vi "Fourier Transform Open VI Final.vi"() -> ()   [LabVIEW 2021]
uses:
  <vilib>/Analysis/4window.llb/windowTd.ctl
  <vilib>/Analysis/4window.llb/Hanning Window (DBL).vi
  <vilib>/Analysis/4window.llb/AllCosWindow (DBL).vi
  <vilib>/Utility/file.llb/Read Delimited Spreadsheet (DBL).vi
  <vilib>/Analysis/2dsp.llb/Zero Padder (DBL).vi
  <vilib>/measure/maspectr.llb/FFT Spectrum (Mag-Phase) for 1 Chan.vi
  <vilib>/measure/NI_MAPro.lvlib
  <vilib>/Analysis/NI_AALPro.lvlib
panel:
  out "Transient":cluster{dbl[], "magnitude":dbl[]}(graph)
  in  "Max m/z Value":dbl=5000.0
  in  "Zero Paddings":i32
  out "Mass Spectrum":cluster{dbl[], "magnitude":dbl[]}(graph)
  out "Mass Calibration Factor":dbl
  out "Frequency (Hz)":dbl
  in  "File Path":path
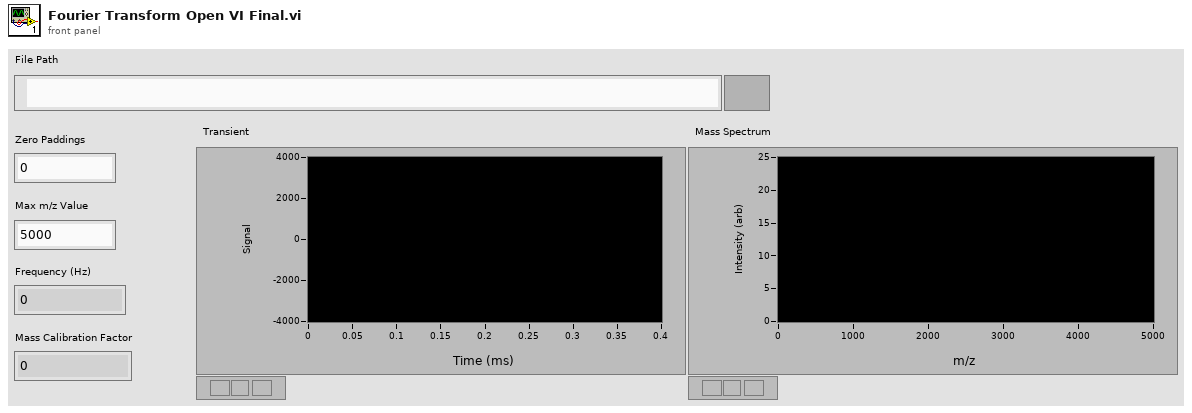
[diagram p1: front panel]
types:
  T1 = typedef "NI_AALPro.lvlib/windowTd.ctl" = u32
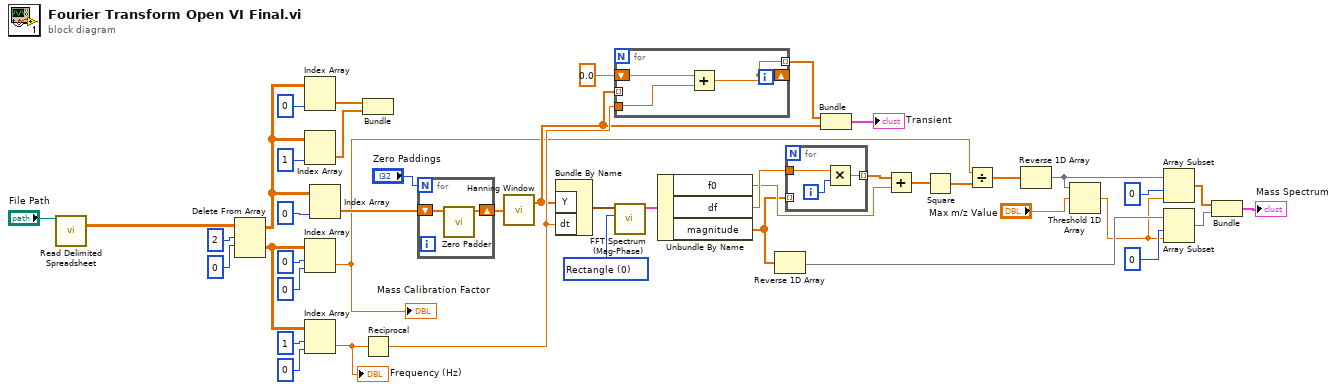
[diagram p0: block diagram]
diagram:
  w26 = T1 0 items=["Rectangle"=0, "Hanning"=1, "Hamming"=2, "Blackman-Harris"=3, "Exact Blackman"=4, "Blackman"=5, "Flat Top"=6, "4 Term B-Harris "=7, "7 Term B-Harris"=8, "Low Sidelobe"=9, "Blackman Nuttall"=11, "Triangle"=30, "Bartlett-Hanning"=31, "Bohman"=32, "Parzen"=33, "Welch"=34, "Kaiser"=60, "Dolph-Chebyshev"=61, "Gaussian"=62] ("window")
  n1 = call-poly <vilib>:"Read Delimited Spreadsheet.vi"("file path (dialog if empty)"="File Path") -> ("all rows"=w43:dbl[][])  [unwired: 9 in, 5 out]
  n2 = Delete From Array(array=w43, length=2, index (row)=0) -> (deleted portion=w39:dbl[][], array with subset deleted=w13:dbl[][])  [unwired: 1 in]
  n3 = Index Array(array=w13, index (col)=0 ("disabled index (col)")) -> (element=w10:dbl[])  [unwired: 1 in]
  n4 = Index Array(array=w13, index (col)=1 ("disabled index (col)")) -> (element=w11:dbl[])  [unwired: 1 in]
  n5 = Index Array(array=w39, index (row)=0, index (col)=0 ("disabled index (col)")) -> (element=w1:dbl)
  "Mass Calibration Factor" <- w1
  n6 = Index Array(array=w39, index (row)=1, index (col)=0 ("disabled index (col)")) -> (element=w29:dbl)
  "Frequency (Hz)" <- w29
  n7 = Index Array(array=w13, index (col)=0 ("disabled index (col)")) -> (element=w32:dbl[])  [unwired: 1 in]
  n8 = Bundle("all rows"=w10, "all rows"=w11) -> ()  [unwired: 1 in, 1 out]
  n9 = Reciprocal(x=w29) -> (1/x=w8:dbl)
  n10 = for {
    N: "Zero Paddings" -> [_]
    shift-right: [w45] -> w31
    shift-left: w32 -> [w46]
    n11 = call-poly <vilib>:"Zero Padder.vi"("Input Array"=w46) -> ("Zero Padded Array"=w45:dbl[])  [unwired: 10 in]
  }
  n12 = call-poly <vilib>:"Hanning Window.vi"("X"=w31) -> ("Windowed X"=w5:dbl[])  [unwired: 1 out]
  n13 = Bundle By Name("Y"=w5, "dt"=w8) -> (w25:waveform(dbl))  [unwired: 1 in]
  n14 = for {
    tunnel: w5 -> [_] mode=indexing
    tunnel: w8 -> [w47]
    shift-right: [w48] -> _
    shift-left: 0.0 -> [w49]
    tunnel: [w48] -> w6 mode=indexing
    n15 = Add(x=w49, y=w47) -> (x+y=w48:dbl)
  }
  n16 = call-poly <vilib>:"FFT Spectrum (Mag-Phase).vi"("window"=w26, "time signal"=w25) -> ("magnitude"=w24:cluster{"f0":dbl, "df":dbl, "magnitude":dbl[]})  [unwired: 5 in, 4 out]
  n17 = Unbundle By Name(w24) -> ("f0"=w35:dbl, "df"=w37:dbl, "magnitude"=w9:dbl[])
  n18 = Reverse 1D Array(array=w9) -> (reversed array=w22:dbl[])
  n19 = for {
    tunnel: w9 -> [_] mode=indexing
    tunnel: w37 -> [w52]
    tunnel: [w51] -> w36 mode=indexing
    i -> [w50]
    n20 = Multiply(x=w52, y=w50) -> (x*y=w51:dbl)
  }
  n21 = Bundle(w6, "Windowed X"=w5) -> (→"Transient":cluster{dbl[], "Windowed X":dbl[]})  [unwired: 1 in]
  n22 = Add(x=w36, y=w35) -> (x+y=w34:dbl[])
  n23 = Square(x=w34) -> (x^2=w33:dbl[])
  n24 = Divide(x=w1, y=w33) -> (x/y=w23:dbl[])
  n25 = Reverse 1D Array(array=w23) -> (reversed array=w20:dbl[])
  n26 = Threshold 1D Array(2:"Max m/z Value", 3:w20) -> (0:w19:dbl)  [unwired: 1 in]
  n27 = Array Subset(array=w20, index=0, length=w19) -> (w17:dbl[])
  n28 = Array Subset(array=w22, index=0 ("length"), length=w19) -> (w16:dbl[])
  n29 = Bundle(w17, w16) -> (→"Mass Spectrum":cluster{dbl[], dbl[]})  [unwired: 1 in]
